vi "get_type.vi"(8 "error in (no error)":errorcluster, 11 "DataFrame in":refnum<class "DataFrame.lvclass">) -> (0 "error out":errorcluster, 2 "type":u8, 3 "DataFrame out":refnum<class "DataFrame.lvclass">)   [LabVIEW 2017, in "DataFrame.lvclass"]
uses:
  DataFrame.lvclass
  DataFrame.lvclass/DataFrame.ctl
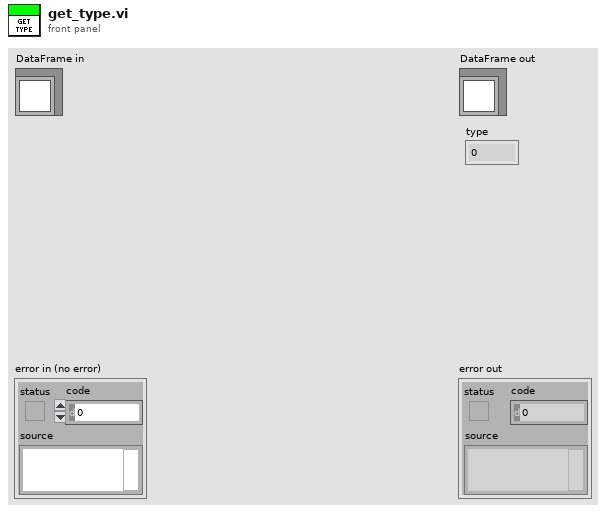
[diagram p1: front panel]
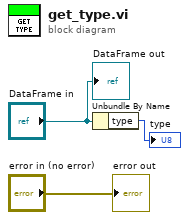
[diagram p0: block diagram]
diagram:
  n1 = Unbundle By Name("DataFrame in") -> ("type"=→"type":u8)
  "error out" <- "error in (no error)"
  "DataFrame out" <- "DataFrame in"
